vi "Stop Spike.vi"(11 "Execute?":bool) -> (3 "Done":bool)   [LabVIEW 2012]
uses:
  <vilib>/Rock Robotics/WPI/Relay/WPI_RelayValue.ctl
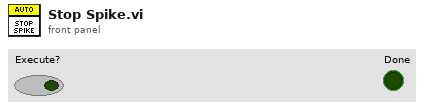
[diagram p1: front panel]
types:
  T1 = typedef "WPI_RelayDevRef.ctl" = cluster{"DevStatus":errorcluster, "Relay Channel":T2, "Digital Module":T3, "Relay Direction":T4}
  T2 = typedef "FPGA_DIORelayChannel.ctl" = enum8{"Relay 1", "Relay 2", "Relay 3", "Relay 4", "Relay 5", "Relay 6", "Relay 7", "Relay 8", "Invalid"}
  T3 = typedef "FPGA_TypedefDigitalModule.ctl" = enum16{"Digital Module 1", "Digital Module 2"}
  T4 = typedef "WPI_RelayDirection.ctl" = enum16{"Both directions", "Forward only", "Reverse only"}
  T5 = typedef "WPI_RelayValue.ctl" = enum16{"Off", "On", "Forward", "Reverse"}
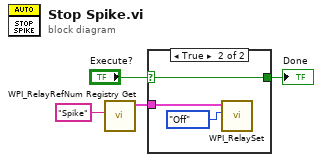
[diagram p0: block diagram]
diagram:
  n1 = call <vilib>:"WPI_RelayRefNum Registry Get.vi"("refnum name"="Spike") -> ("RelayDevRef"=w2:T1)  [unwired: 9 in, 1 out]
  n2 = case shown="True" "Execute?" {
    selector: "Execute?" -> [w5 w8]
    tunnel: [w5 w8] -> w3
    tunnel: w2 -> [_ w6]
    frame False {
    }
    frame True {
      n3 = call <vilib>:"WPI_RelaySet.vi"("RelayValue"=WPI_RelayValue."Off", "RelayDevRef"=w6) -> ()  [unwired: 8 in, 2 out]
    }
  }
  "Done" <- w3
